vi "LDO Bit Status Write.vi"(0 "LDO Control Input":T1 {"Timing"."Absolute Time" format="%<%H:%M:%S%3u>t"; "Timing"."Display Time" format="%#.20f"; "Timing"."Test Time Ref" format="%#.20f"; "Timing"."Precondition Time Ref" format="%#.20f"; "Timing"."First Call Time Ref" format="%#.20f"}, 5 "Condition A":bool, 7 "Condition B":bool, 9 "Condition C":bool, 11 "error in":errorcluster, 12 "Stop Test":bool) -> (4 "Bit Status":string[][](array[string]), 15 "error out":errorcluster)   [LabVIEW 2023]
uses:
  Modbus/Modbus LDO Control.ctl
  Modbus/Modbus Timing.ctl
  <vilib>/Utility/miscctls.llb/LVDateTimeRec.ctl
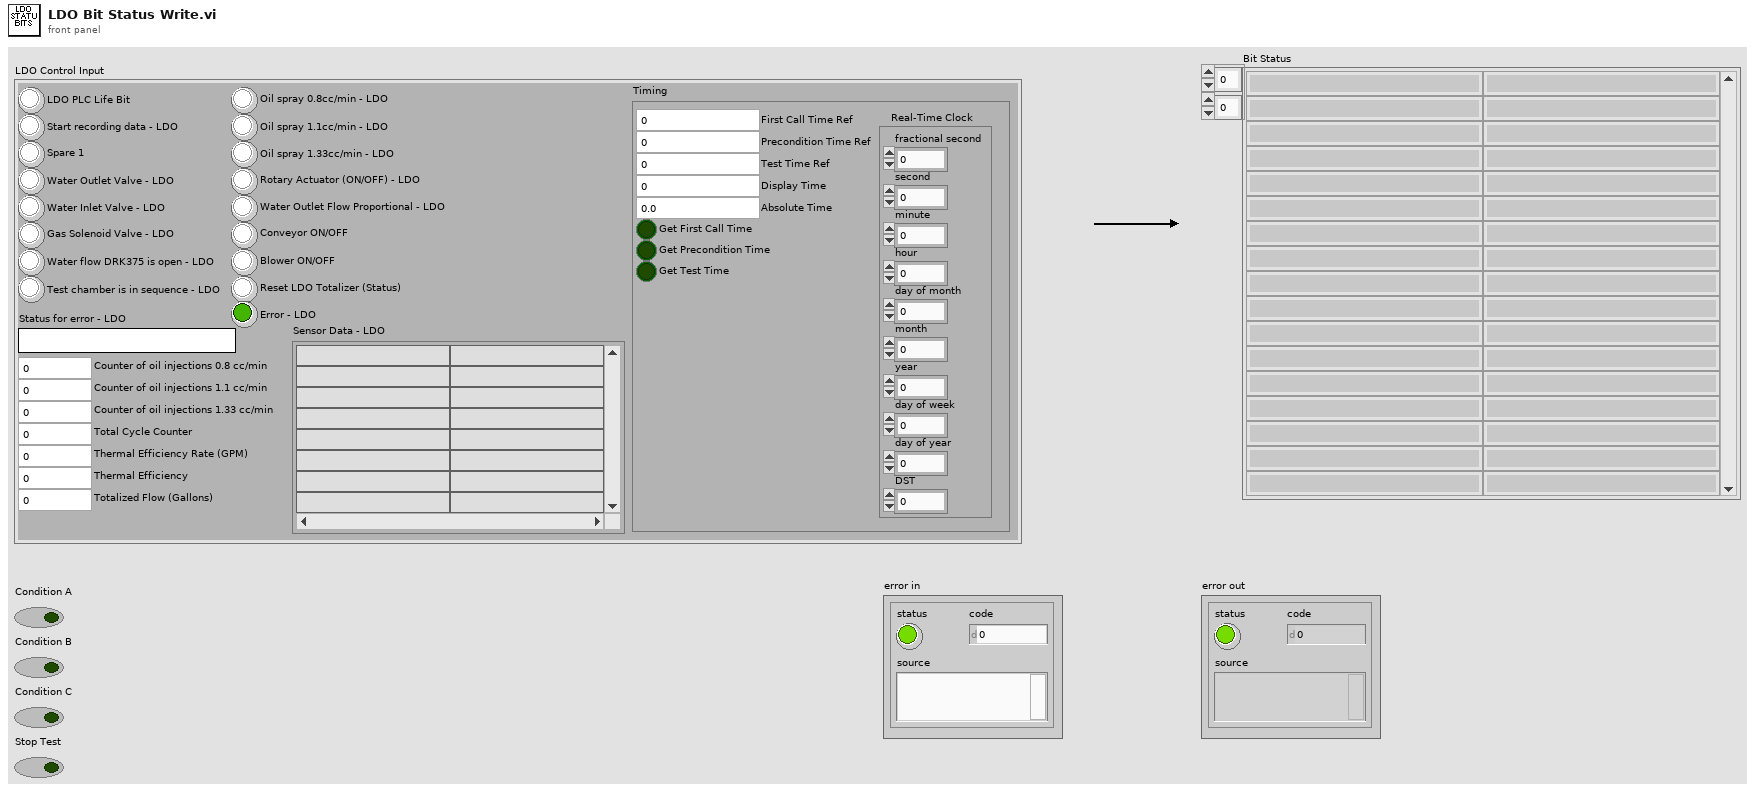
[diagram p1: front panel]
types:
  T1 = typedef "Modbus LDO Control.ctl" = cluster{"LDO PLC Life Bit":bool, "Start recording data - LDO":bool, "Spare 1":bool, "Water Outlet Valve - LDO":bool, "Water Inlet Valve - LDO":bool, "Gas Solenoid Valve - LDO":bool, "Water flow DRK375 is open - LDO":bool, "Test chamber is in sequence - LDO":bool, "Oil spray 0.8cc/min - LDO":bool, "Oil spray 1.1cc/min - LDO":bool, "Oil spray 1.33cc/min - LDO":bool, "Rotary Actuator (ON/OFF) - LDO":bool, "Water Outlet Flow Proportional - LDO":bool, "Conveyor ON/OFF":bool, "Blower ON/OFF":bool, "Reset LDO Totalizer (Status)":bool, "Status for error - LDO":string, "Error - LDO":bool, "Sensor Data - LDO":string[][], "Thermal Efficiency Rate (GPM)":dbl, "Thermal Efficiency":dbl, "Totalized Flow (Gallons)":dbl, "Counter of oil injections 1.33 cc/min":u16, "Total Cycle Counter":u16, "Counter of oil injections 1.1 cc/min":u16, "Counter of oil injections 0.8 cc/min":u16, "Timing":T2}
  T2 = typedef "Modbus Timing.ctl" = cluster{"First Call Time Ref":dbl, "Precondition Time Ref":dbl, "Test Time Ref":dbl, "Get First Call Time":bool, "Get Precondition Time":bool, "Get Test Time":bool, "Display Time":dbl, "Real-Time Clock":T3, "Absolute Time":dbl}
  T3 = typedef "LVDateTimeRec.ctl" = cluster{"fractional second":dbl, "second":i32, "minute":i32, "hour":i32, "day of month":i32, "month":i32, "year":i32, "day of week":i32, "day of year":i32, "DST":i32}
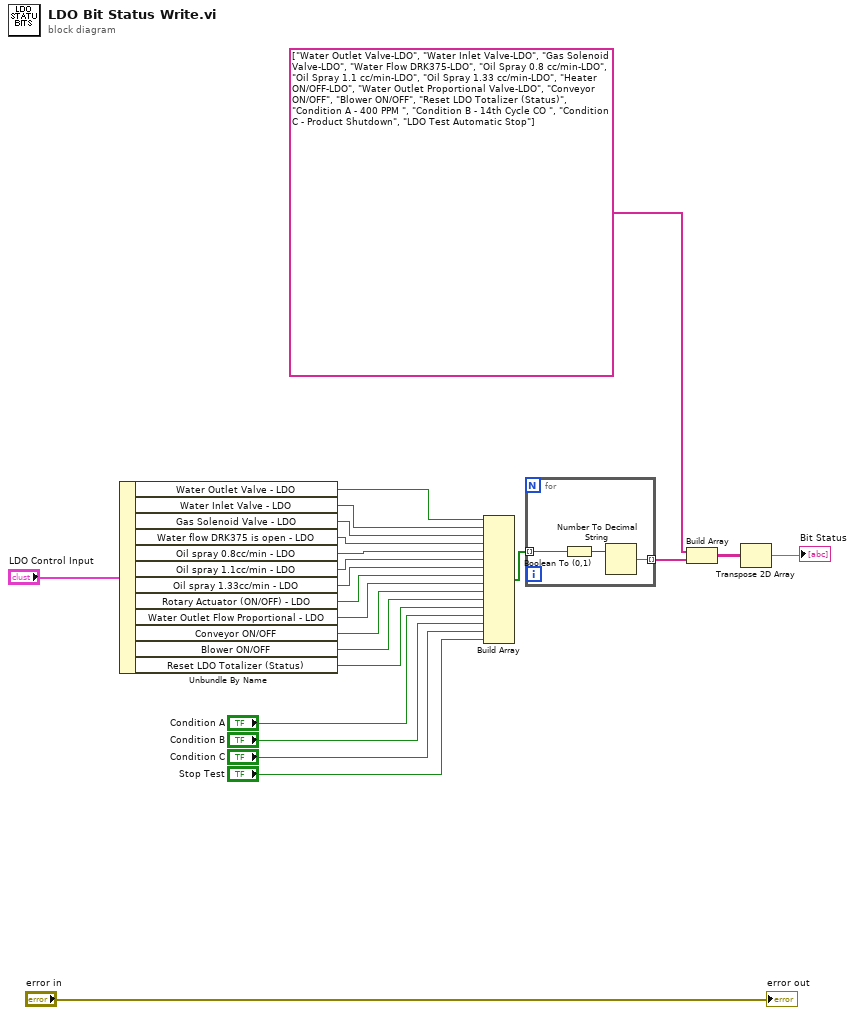
[diagram p0: block diagram]
diagram:
  n1 = Unbundle By Name("LDO Control Input") -> ("Water Outlet Valve - LDO"=w22:bool, "Water Inlet Valve - LDO"=w21:bool, "Gas Solenoid Valve - LDO"=w20:bool, "Water flow DRK375 is open - LDO"=w19:bool, "Oil spray 0.8cc/min - LDO"=w18:bool, "Oil spray 1.1cc/min - LDO"=w17:bool, "Oil spray 1.33cc/min - LDO"=w16:bool, "Rotary Actuator (ON/OFF) - LDO"=w15:bool, "Water Outlet Flow Proportional - LDO"=w14:bool, "Conveyor ON/OFF"=w7:bool, "Blower ON/OFF"=w6:bool, "Reset LDO Totalizer (Status)"=w5:bool)
  n2 = Build Array(w22, w21, w20, w19, w18, w17, w16, w15, w14, w7, w6, w5, "Condition A", "Condition B", "Condition C", "Stop Test") -> (w13:bool[])
  n3 = for {
    tunnel: w13 -> [w25] mode=indexing
    tunnel: [w24] -> w12 mode=indexing
    n4 = Boolean To (0,1)(Boolean=w25) -> (0, 1=w26:i16)
    n5 = Number To Decimal String(number=w26) -> (decimal integer string=w24:string)  [unwired: 1 in]
  }
  n6 = Build Array(string[] ["Water Outlet Valve-LDO", "Water Inlet Valve-LDO", "Gas Solenoid Valve-LDO", "Water Flow DRK375-LDO", "Oil Spray 0.8 cc/min-LDO", "Oil Spray 1.1 cc/min-LDO", "Oil Spray 1.33 cc/min-LDO", "Heater ON/OFF-LDO", "Water Outlet Proportional Valve-LDO", "Conveyor ON/OFF", "Blower ON/OFF", "Reset LDO Totalizer (Status)", "Condition A - 400 PPM ", "Condition B - 14th Cycle CO ", "Condition C - Product Shutdown", "LDO Test Automatic Stop"], w12) -> (w10:string[][])
  n7 = Transpose 2D Array(2D array=w10) -> (transposed array=→"Bit Status":string[][])
  "error out" <- "error in"
